vi "Reload Data Type Information Collection.vi"(8 "error in (no error)":errorcluster, 11 "TwinCAT ADS in":refnum<class "TwinCAT ADS.lvclass">) -> (0 "error out":errorcluster, 3 "TwinCAT ADS out":refnum<class "TwinCAT ADS.lvclass">)   [LabVIEW 2018, in "TwinCAT ADS.lvclass"]
uses:
  TwinCAT ADS.lvclass
  TwinCAT ADS.lvclass/TwinCAT ADS.ctl
  TwinCAT.Ads
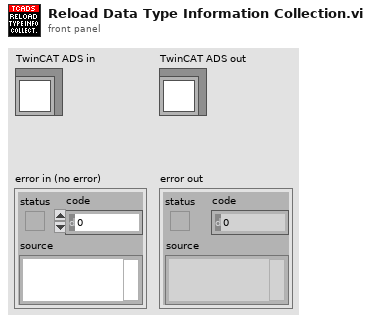
[diagram p1: front panel]
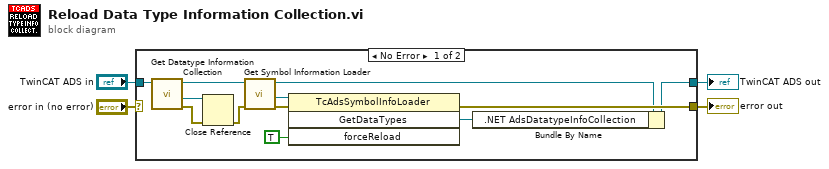
[diagram p0: block diagram]
diagram:
  n1 = case shown="No Error" "error in (no error)" {
    selector: "error in (no error)" -> [_ w18]
    tunnel: [w16 w18] -> w3
    tunnel: [w11 w17] -> w1
    tunnel: "TwinCAT ADS in" -> [w9 w17]
    frame No Error {
      n2 = call "Get Datatype Information Collection.vi"("TwinCAT ADS in"=w9) -> ("error out"=w7:errorcluster, ".NET AdsDatatypeInfoCollection"=w6:refnum<k24>, "TwinCAT ADS out"=w8:refnum<class "TwinCAT ADS.lvclass">)  [unwired: 8 in]
      n3 = Close Reference(reference=w6, error in (no error)=w7) -> (error out=w5:errorcluster)
      n4 = call "Get Symbol Information Loader.vi"("error in (no error)"=w5, "TwinCAT ADS in"=w8) -> ("error out"=w15:errorcluster, ".NET AdsSymbolInfoLoader"=w14:refnum<k24>, "TwinCAT ADS out"=w12:refnum<class "TwinCAT ADS.lvclass">)  [unwired: 7 in]
      n5 = invoke class="TcAdsSymbolInfoLoader" method="GetDataTypes"(reference=w14, error in=w15, "forceReload"=TRUE) -> (error out=w16:errorcluster, "GetDataTypes"=w10:refnum<k24>)  [unwired: 1 in, 2 out]
      n6 = Bundle By Name(cluster=w12, ".NET AdsDatatypeInfoCollection"=w10) -> (w11:refnum<class "TwinCAT ADS.lvclass">)
    }
    frame Error {
    }
  }
  "error out" <- w3
  "TwinCAT ADS out" <- w1
